vi "whileState.vi"(8 "error in (no error)":errorcluster, 11 "User-Defined in":refnum<class "user-defined-state.lvclass">) -> (0 "error out":errorcluster, 1 "Done?":bool, 2 "next state":refnum<class "state.lvclass">, 3 "User-Defined out":refnum<class "user-defined-state.lvclass">)   [LabVIEW 2020, in "eos.lvlib" / "user-defined-state.lvclass"]
uses:
  user-defined-state.lvclass
  interfaces/state/state.lvclass
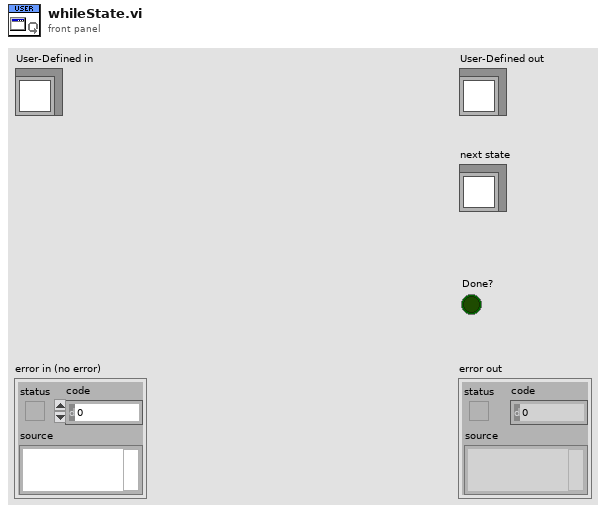
[diagram p1: front panel]
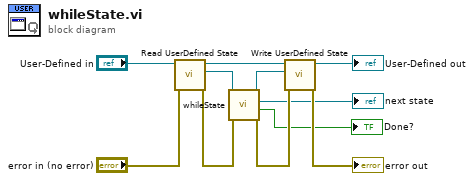
[diagram p0: block diagram]
diagram:
  n1 = call "Read UserDefined State.vi"("error in (no error)"="error in (no error)", "user-defined-state in"="User-Defined in") -> ("error out"=w9:errorcluster, "state"=w6:refnum<class "state.lvclass">, "user-defined-state out"=w8:refnum<class "user-defined-state.lvclass">)  [unwired: 7 in]
  n2 = call-dynamic "whileState.vi"("error in (no error)"=w9, "state in"=w6) -> ("error out"=w4:errorcluster, "Done?"=→"Done?":bool, "next state"=→"next state":refnum<class "state.lvclass">, "state out"=w5:refnum<class "state.lvclass">)  [unwired: 6 in]
  n3 = call "Write UserDefined State.vi"("error in (no error)"=w4, "state"=w5, "user-defined-state in"=w8) -> ("error out"=→"error out":errorcluster, "user-defined-state out"=→"User-Defined out":refnum<class "user-defined-state.lvclass">)  [unwired: 7 in]
